vi "Zero AO Amplitudes.vi"(8 "error in (no error)":errorcluster, 11 "Instrument.DAQ in":refnum<class "Instrument.DAQ.lvclass">) -> (0 "error out":errorcluster, 2 "Saved Amplitudes":dbl[](array[numeric]), 3 "Instrument.DAQ out":refnum<class "Instrument.DAQ.lvclass">)   [LabVIEW 2019, in "Instrument.Lockin.lvlib" / "Instrument.DAQ.lvclass"]
uses:
  Instrument.DAQ.lvclass
  Instrument.DAQ.lvclass/Instrument.DAQ.ctl
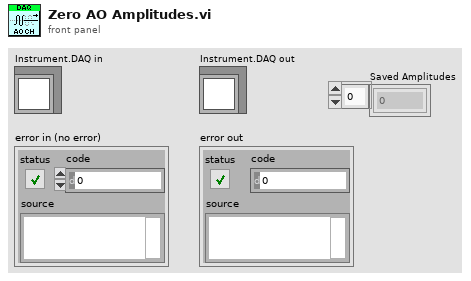
[diagram p1: front panel]
types:
  T1 = typedef "Instrument.Lockin.lvlib/Instrument.DAQ.lvclass/AO.Channel--Cluster--Array.ctl" = T2[]
  T2 = typedef "Instrument.Lockin.lvlib/Instrument.DAQ.lvclass/AO.Channel--Cluster.ctl" = cluster{"Enable?":bool, "Channel":i32, "Amplitude":dbl, "Offset":dbl, "Frequency":dbl, "Phase":dbl, "Function":T3, "Sweeping?":bool, "Limit AC":bool, "Limit DC?":bool, "Duty Cycle":bool}
  T3 = typedef "Instrument.Lockin.lvlib/Instrument.DAQ.lvclass/AO.Channel.Function--Enum.ctl" = enum16{"sine", "square", "triangle", "saw"}
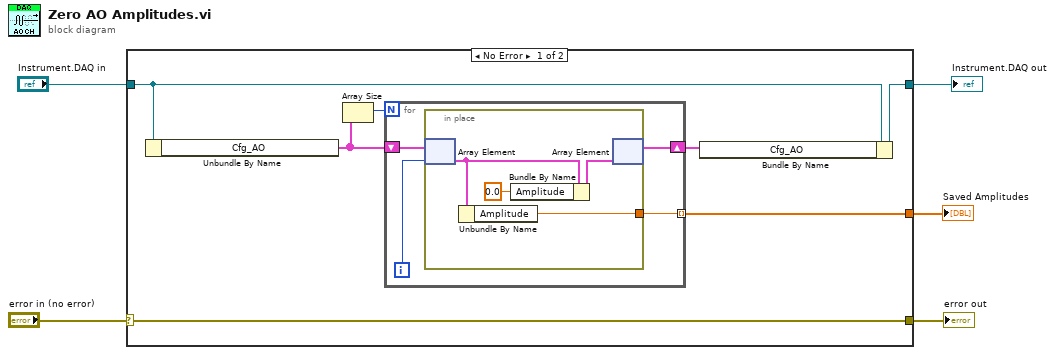
[diagram p0: block diagram]
diagram:
  n1 = case shown="No Error" "error in (no error)" {
    selector: "error in (no error)" -> [w6 w22]
    tunnel: [w11 w21] -> w5
    tunnel: "Instrument.DAQ in" -> [w10 w21]
    tunnel: [w7 _] -> w3
    tunnel: [w6 w22] -> w1
    frame No Error {
      n2 = Unbundle By Name(w10) -> ("Cfg_AO"=w9:T1)
      n3 = Array Size(array=w9) -> (size(s)=w8:i32)
      n4 = for {
        N: w8 -> [_]
        tunnel: [w16] -> w7 mode=indexing
        shift-right: [w13] -> w12
        shift-left: w9 -> [w15]
        i -> [w14]
        n5 = in-place {
          in-place-border: [w20] -> w16
          n6 = in-place-array #1(w15, w14) -> (w18:T2)
          n7 = Unbundle By Name(w18) -> ("Amplitude"=w20:dbl)
          n8 = Bundle By Name(cluster=w18, "Amplitude"=0.0) -> (w17:T2)
          n9 = in-place-array #1(w17) -> (w13:T1)  [unwired: 1 out]
        }
      }
      n10 = Bundle By Name(cluster=w10, "Cfg_AO"=w12) -> (w11:refnum<class "Instrument.DAQ.lvclass">)
    }
    frame Error {
    }
  }
  "error out" <- w1
  "Instrument.DAQ out" <- w5
  "Saved Amplitudes" <- w3
